vi "QMH_ICR_Create_User_Exit_Event.vi"(8 "error in (no error)":errorcluster caption="entrée d'erreur (pas d'erreur)") -> (0 "error out":errorcluster caption="sortie d'erreur", 2 "User Exit Event":refnum<user-event>, 3 "Refnum register for events":refnum<event-registration>)   [LabVIEW 2015]
panel:
  out "Refnum d'abonnement à des événements":refnum<event-registration>
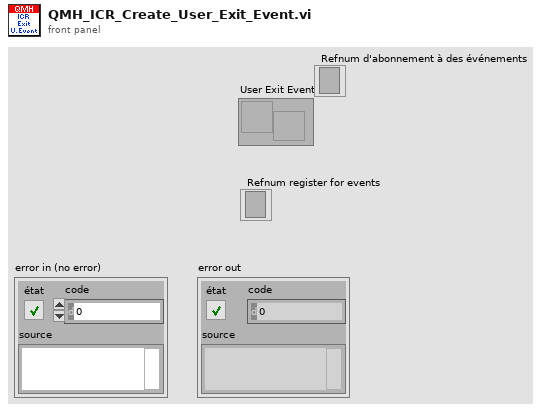
[diagram p1: front panel]
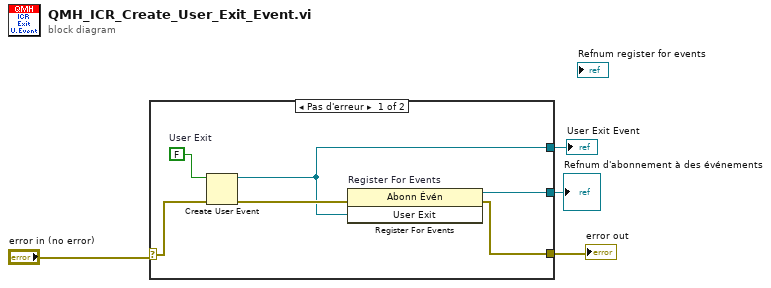
[diagram p0: block diagram]
diagram:
  n1 = case shown="Pas d'erreur" "error in (no error)" {
    selector: "error in (no error)" -> [w8 w11]
    tunnel: [w5 _] -> w1
    tunnel: [w9 _] -> w2
    tunnel: [w7 w11] -> w3
    frame No Error {
      w6 = FALSE  # User Exit
      n2 = Create User Event(user event datatype=w6, error in=w8) -> (user event=w9:refnum<user-event>, error out=w10:errorcluster)
      n3 = register-events "Register For Events"(error in=w10, w9) -> (reference out=w5:refnum<event-registration>, error out=w7:errorcluster)  [unwired: 1 in]
    }
    frame Error {
    }
  }
  "error out" <- w3
  "User Exit Event" <- w2
  "Refnum d'abonnement à des événements" <- w1
